vi "terminate.vi"(8 "error in (no error)":errorcluster, 11 "StreamingBase in":refnum<class "StreamingBase.lvclass">) -> (0 "error out":errorcluster, 3 "StreamingBase out":refnum<class "StreamingBase.lvclass">)   [LabVIEW 2011, in "StreamingBase.lvclass"]
uses:
  StreamingBase.lvclass
  StreamingBase.lvclass/StreamingBase.ctl
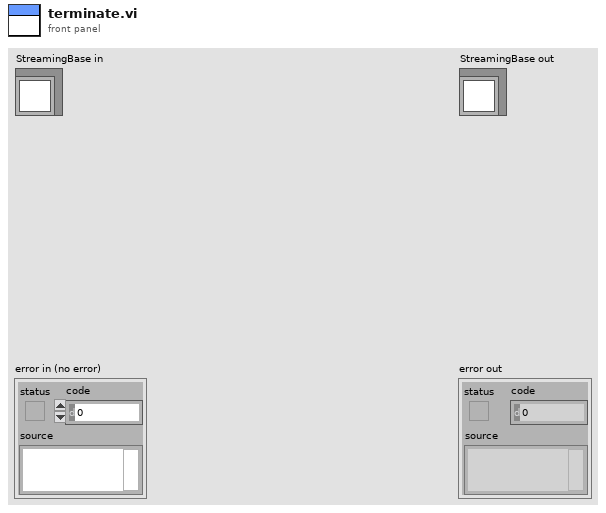
[diagram p1: front panel]
types:
  T1 = typedef "StreamingBase.lvclass/observer_cluster.ctl" = cluster{"writer endpoint":refnum<k21>, "reader endpoint":refnum<k21>}
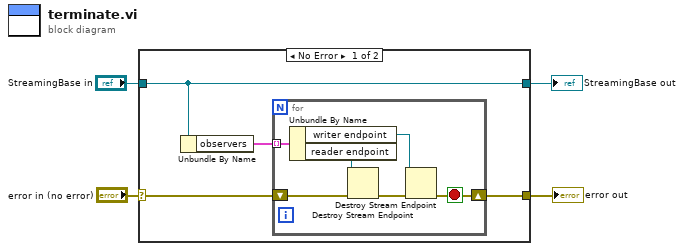
[diagram p0: block diagram]
diagram:
  n1 = case shown="No Error" "error in (no error)" {
    selector: "error in (no error)" -> [w6 w16]
    tunnel: [w5 w16] -> w3
    tunnel: [w8 w15] -> w1
    tunnel: "StreamingBase in" -> [w8 w15]
    frame No Error {
      n2 = Unbundle By Name(w8) -> ("observers"=w7:T1[])
      n3 = for {
        tunnel: w7 -> [w14] mode=indexing
        shift-right: [w9] -> w5
        shift-left: w6 -> [w13]
        stop <- w9 stop-if-true
        n4 = Unbundle By Name(w14) -> ("writer endpoint"=w11:refnum<k21>, "reader endpoint"=w12:refnum<k21>)
        n5 = Destroy Stream Endpoint(8:w13, 11:w12) -> (0:w10:errorcluster)
        n6 = Destroy Stream Endpoint(8:w10, 11:w11) -> (0:w9:errorcluster)
      }
    }
    frame Error {
    }
  }
  "error out" <- w3
  "StreamingBase out" <- w1
